vi "PlotStep.vi"(7 "StepPlotData":dbl[][][][][](array[numeric]), 9 "index":u32[](array[numeric]), 10 "ctlPlot":T1, 11 "StepTVEData":dbl[][][][][](array[numeric])) -> (2 "StepPlot":cluster{"Array":dbl[], "Array":dbl[]}(graph), 3 "StepTVE":cluster{"Array":dbl[], "Array":dbl[]}(graph))   [LabVIEW 2014]
uses:
  typedef/ctlPlot.ctl
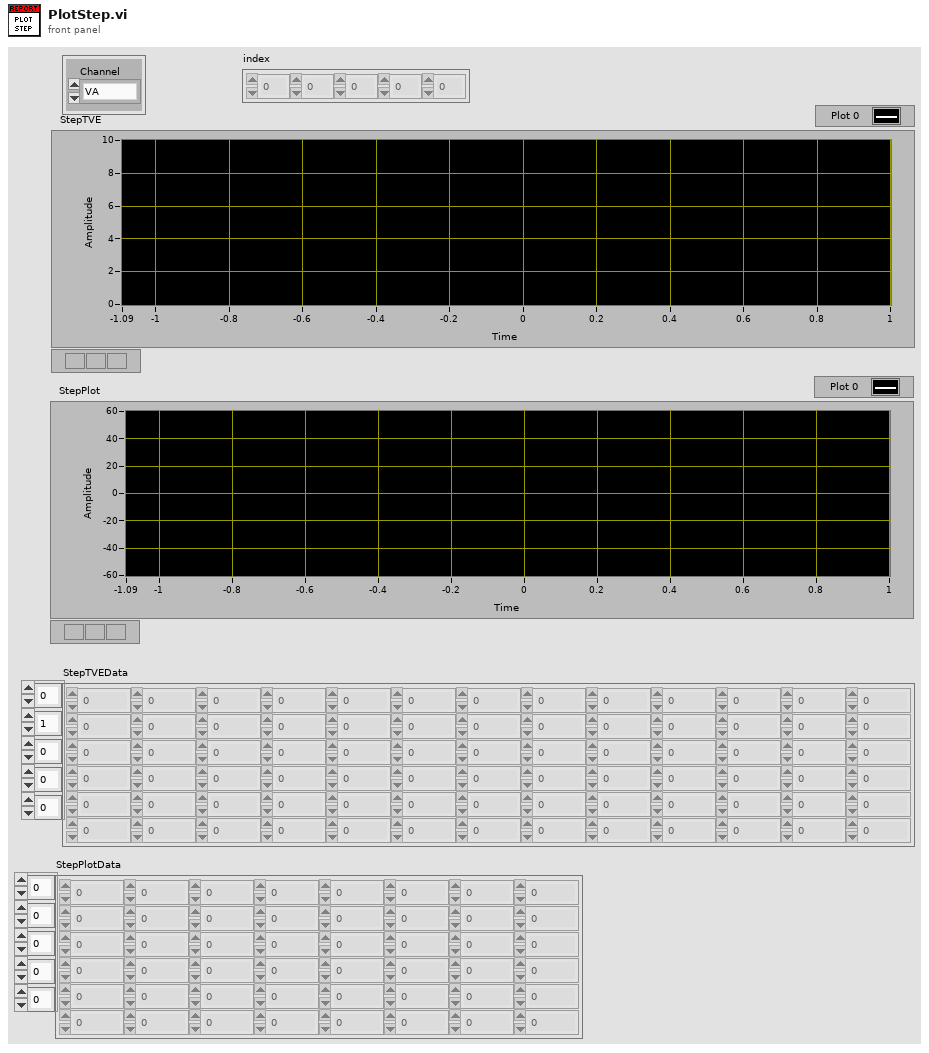
[diagram p1: front panel]
types:
  T1 = typedef "ctlPlot.ctl" = cluster{"Channel":enum16{"VA", "VB", "VC", "V+", "IA", "IB", "IC", "I+", "FREQ", "ROCOF"}, "Parameter":enum16{"TVE", "ME", "PE"}}
  T2 = enum16{"VA", "VB", "VC", "V+", "IA", "IB", "IC", "I+", "FREQ", "ROCOF"}
  T3 = cluster{"StepTVEData":dbl[], "StepPlotData":dbl[]}
  T4 = cluster{"StepTVEData":dbl[], "StepTVEData":dbl[]}
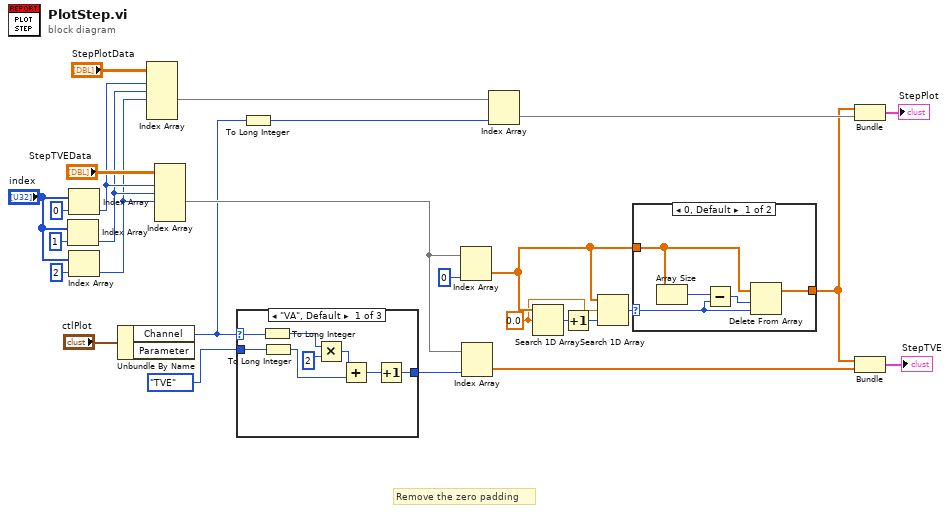
[diagram p0: block diagram]
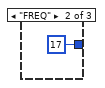
[diagram p3: hidden frame]
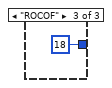
[diagram p4: hidden frame]
diagram:
  w3 = 0.0 ("element")
  # "Remove the zero padding"
  n1 = Index Array(array="index", index=1) -> (element=w14:u32)
  n2 = Index Array(array="index", index=0) -> (element=w15:u32)
  n3 = Index Array(array="index", index=2) -> (element=w13:u32)
  n4 = Unbundle By Name("ctlPlot") -> ("Channel"=w9:T2)  [unwired: 1 out]
  n5 = Index Array(array="StepPlotData", index (dim 0)=w15, index (dim 1)=w14, index (dim 2)=w13) -> (element=w12:dbl[][])  [unwired: 2 in]
  n6 = Index Array(array="StepTVEData", index (dim 0)=w15, index (dim 1)=w14, index (dim 2)=w13) -> (element=w23:dbl[][])  [unwired: 2 in]
  n7 = case shown="\"VA\", Default" w9 {
    selector: w9 -> [w28 _ _]
    tunnel: enum16{"TVE", "ME", "PE"}."TVE" ("Parameter") -> [w33 _ _]
    tunnel: [w29 17 18] -> w18
    frame "VA", Default {
      n8 = To Long Integer(number=w28) -> (32bit integer=w31:i32)
      n9 = To Long Integer(number=w33) -> (32bit integer=w32:i32)
      n10 = Multiply(x=w31, y=2) -> (x*y=w35:i32)
      n11 = Add(x=w35, y=w32) -> (x+y=w30:i32)
      n12 = Increment(x=w30) -> (x+1=w29:i32)
    }
    frame "FREQ" {
    }
    frame "ROCOF" {
    }
  }
  n13 = To Long Integer(number=w9) -> (32bit integer=w8:i32)
  n14 = Index Array(array=w23, index (col)=0 ("disabled index (row)")) -> (element=w7:dbl[])  [unwired: 1 in]
  n15 = Index Array(array=w23, index (col)=w18) -> (element=w24:dbl[])  [unwired: 1 in]
  n16 = Index Array(array=w12, index (col)=w8) -> (element=w10:dbl[])  [unwired: 1 in]
  n17 = Search 1D Array(1D array=w7, element=w3) -> (index of element=w4:i32)  [unwired: 1 in]
  n18 = Increment(x=w4) -> (x+1=w1:i32)
  n19 = Search 1D Array(1D array=w7, element=w3, start index (0)=w1) -> (index of element=w2:i32)
  n20 = case shown="0, Default" w2 {
    selector: w2 -> [w38 _]
    tunnel: w7 -> [w42 w43]
    tunnel: [w41 w43] -> w6
    frame 0, Default {
      n21 = Array Size(array=w42) -> (size(s)=w40:i32)
      n22 = Subtract(x=w40, y=w38) -> (x-y=w39:i32)
      n23 = Delete From Array(array=w42, length=w39, index=w38) -> (array with subset deleted=w41:dbl[])  [unwired: 1 out]
    }
    frame -1 {
      # "There is no 0 padding"
    }
  }
  n24 = Bundle("StepTVEData"=w6, "StepPlotData"=w10) -> (→"StepPlot":T3)  [unwired: 1 in]
  n25 = Bundle("StepTVEData"=w6, "StepTVEData"=w24) -> (→"StepTVE":T4)  [unwired: 1 in]
